vi "Lifter enc fun.vi"(6 "intake input":dbl, 8 "error in (no error)":errorcluster, 9 "butten 5":bool, 10 "butten 4":bool, 11 "CAN Talon SRX Ref":T1={"DeviceStatus"={"status"=FALSE, "code"=0, "source"=""}, "Type"=enum."PWM", "PWM"={"PWM Channel"=enum."Invalid", "DeadBand"={"Name"="", "maxPositivePwm"=0, "minPositivePwm"=0, "centerPwm"=0, "maxNegativePwm"=0, "minNegativePwm"=0, "angularRange"=0}}, "CAN"={"Device Number"=0, "Control Mode"=enum."Percent VBus", "Semaphore"=refnum, "Max Vout"=12.0, "TalonSRX Control Mode"=enum."Percent VBus"}, "Invert"=FALSE}) -> (0 "error out":errorcluster, 1 "Intake output":dbl, 2 "Lifter output":dbl, 3 "CAN Talon SRX Ref 2":T1={"DeviceStatus"={"status"=FALSE, "code"=0, "source"=""}, "Type"=enum."PWM", "PWM"={"PWM Channel"=enum."PWM 1", "DeadBand"={"Name"="", "maxPositivePwm"=0, "minPositivePwm"=0, "centerPwm"=0, "maxNegativePwm"=0, "minNegativePwm"=0, "angularRange"=0}}, "CAN"={"Device Number"=0, "Control Mode"=enum."Percent VBus", "Semaphore"=refnum, "Max Vout"=12.0, "TalonSRX Control Mode"=enum."Percent VBus"}, "Invert"=FALSE})   [LabVIEW 2015]
uses:
  <vilib>/Rock Robotics/WPI/MotorControl/WPI_MotorControlDeviceRef.ctl
  <vilib>/Rock Robotics/WPI/MotorControl/WPI_MotorControlType.ctl
  <vilib>/Rock Robotics/SystemInterfaces/DIO/FPGA_DIOPWMChannel.ctl
  <vilib>/Rock Robotics/WPI/PWM/WPI_PWMDeadband.ctl
  <vilib>/Rock Robotics/WPI/CAN/Jaguar/SubVIs/WPI_CANJaguar_ControlMode.ctl
  <vilib>/Rock Robotics/WPI/CAN/TalonSRX/WPI_CANTalonSRX_APIControlMode.ctl
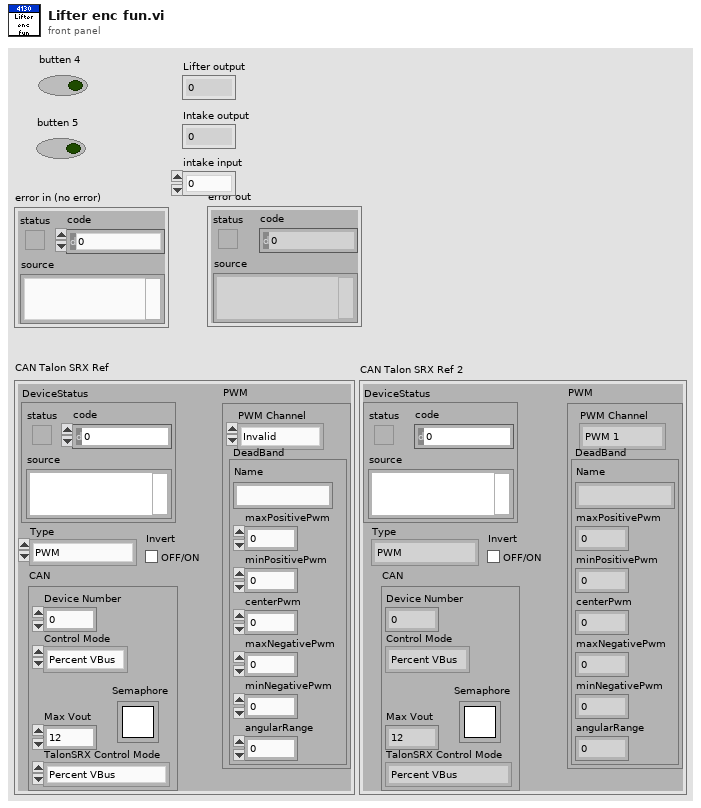
[diagram p1: front panel]
types:
  T1 = typedef "WPI_MotorControlDeviceRef.ctl" = cluster{"DeviceStatus":errorcluster, "Type":T2, "PWM":cluster{"PWM Channel":T3, "DeadBand":T4}, "CAN":cluster{"Device Number":u8, "Control Mode":T5, "Semaphore":T6, "Max Vout":dbl, "TalonSRX Control Mode":T7}, "Invert":bool}
  T2 = typedef "WPI_MotorControlType.ctl" = enum16{"PWM", "CAN", "CANTalonSRX"}
  T3 = typedef "FPGA_DIOPWMChannel.ctl" = enum8{"PWM 0", "PWM 1", "PWM 2", "PWM 3", "PWM 4", "PWM 5", "PWM 6", "PWM 7", "PWM 8", "PWM 9", "PWM MXP 0", "PWM MXP 1", "PWM MXP 2", "PWM MXP 3", "PWM MXP 4", "PWM MXP 5", "PWM MXP 6", "PWM MXP 7", "PWM MXP 8", "PWM MXP 9", "Invalid"}
  T4 = typedef "WPI_PWMDeadband.ctl" = cluster{"Name":string, "maxPositivePwm":i32, "minPositivePwm":i32, "centerPwm":i32, "maxNegativePwm":i32, "minNegativePwm":i32, "angularRange":u16}
  T5 = typedef "WPI_CANJaguar_ControlMode.ctl" = enum8{"Percent VBus", "Current", "Speed", "Position", "Voltage"}
  T6 = typedef "Semaphore RefNum" = refnum<k1>
  T7 = typedef "WPI_CANTalonSRX_APIControlMode.ctl" = enum8{"Percent VBus", "Speed", "Position", "Slave", "Unchanged / Invalid", "Voltage Compensation", "Current", "Motion Profile"}
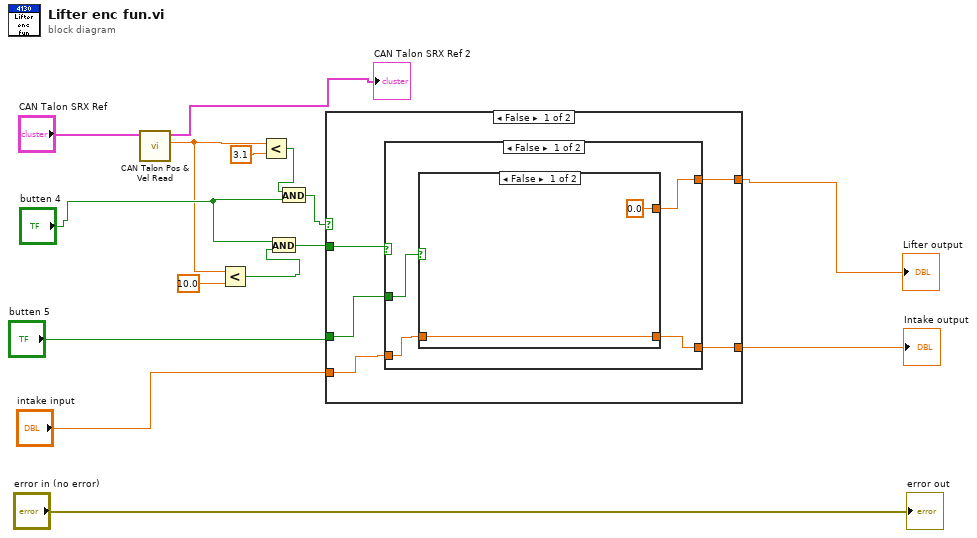
[diagram p0: block diagram]
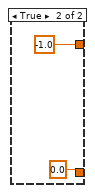
[diagram p2: hidden frame]
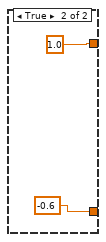
[diagram p3: hidden frame]
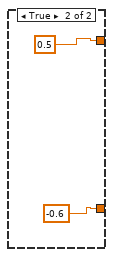
[diagram p4: hidden frame]
diagram:
  n1 = call "CAN Talon Pos & Vel Read.vi"("CAN Talon SRX Ref"="CAN Talon SRX Ref") -> ("Sensor Position"=w5:dbl, "CAN Talon SRX Ref"=→"CAN Talon SRX Ref 2":T1)  [unwired: 6 in, 3 out]
  n2 = Less?(x=w5, y=10.0) -> (x < y?=w1:bool)
  n3 = Less?(x=w5, y=3.1) -> (x < y?=w13:bool)
  n4 = And(x="butten 4", y=w1) -> (x .and. y?=w7:bool)
  n5 = And(x=w13, y="butten 4") -> (x .and. y?=w12:bool)
  n6 = case shown="False" w12 {
    tunnel: w7 -> [w20 _]
    tunnel: [w19 0.5 ("y")] -> w11
    tunnel: [w18 -0.6 ("y")] -> w10
    tunnel: "intake input" -> [w17 _]
    tunnel: "butten 5" -> [w16 _]
    frame False {
      n7 = case shown="False" w20 {
        tunnel: [w23 1.0 ("y")] -> w19
        tunnel: [w21 -0.6 ("y")] -> w18
        tunnel: w17 -> [w22 _]
        tunnel: w16 -> [w24 _]
        frame False {
          n8 = case shown="False" w24 {
            tunnel: [0.0 ("y") -1.0 ("y")] -> w23
            tunnel: w22 -> [w26 _]
            tunnel: [w26 0.0 ("intake input")] -> w21
            frame False {
            }
            frame True {
            }
          }
        }
        frame True {
        }
      }
    }
    frame True {
    }
  }
  "Intake output" <- w10
  "Lifter output" <- w11
  "error out" <- "error in (no error)"
